vi "Andor Camera Temperature.vi"() -> ()   [LabVIEW 2014]
panel:
  out "Andor Camera Temperature":dbl
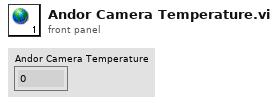
[diagram p1: front panel]
diagram:
